vi "Test Registry Access.vi"() -> ()   [LabVIEW 2011, in "Diamond Universal Driver.lvlib"]
uses:
  Diamond Universal Driver.lvlib
  support/dlls/mm32at.dll
panel:
  out "error out":errorcluster
  out "Boolean array":bool[](array[boolean])
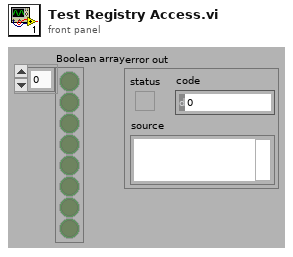
[diagram p1: front panel]
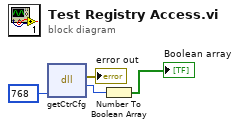
[diagram p0: block diagram]
diagram:
  n1 = dll-call lib="C:/Users/mrichardson/Documents/Web Based Version Control SW/Reusable/Diamond Universal Driver/support/dlls/mm32at.dll" fn="getCtrCfg"("address"=u16 768) -> (error out=→"error out":errorcluster, "cfgOut"=w3:u8)  [unwired: 4 in, 1 out]
  n2 = Number To Boolean Array(number=w3) -> (Boolean array=→"Boolean array":bool[])
